vi "AB_Log_LinkerInfo.vi"(8 "error in (no error)":errorcluster, 10 "linksToInclude":string, 11 "pathsToRead":path[](array[path])) -> (0 "error out":errorcluster)   [LabVIEW 2020]
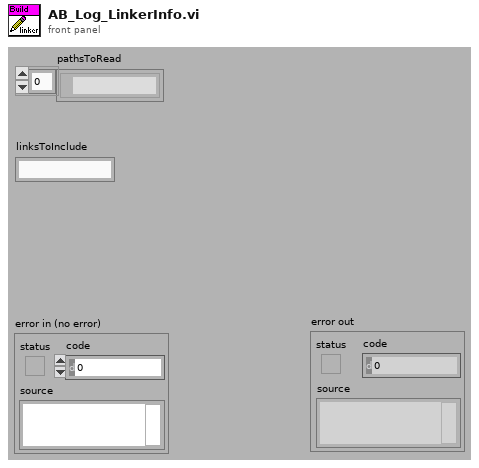
[diagram p1: front panel]
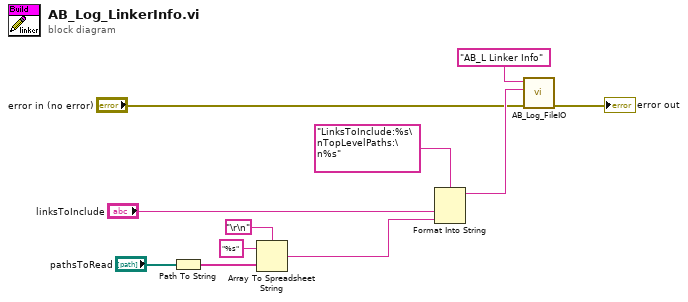
[diagram p0: block diagram]
diagram:
  n1 = Path To String(path="pathsToRead") -> (string=w4:string[])
  n2 = Array To Spreadsheet String(delimiter (Tab)="\r\n", array=w4, 3:"%s" ("format string")) -> (spreadsheet string=w2:string)
  n3 = Format Into String(format string="LinksToInclude:%s\nTopLevelPaths:\n%s", "linksToInclude", w2) -> (resulting string=w10:string)  [unwired: 2 in, 1 out]
  n4 = call <vilib>:"AB_Log_FileIO.vi"("error in (no error)"="error in (no error)", "data"=w10, "newSection"="AB_L Linker Info" ("data")) -> ("error out"=→"error out":errorcluster)  [unwired: 8 in]
